vi "Write Expanded_.vi"(8 "error in (no error)":errorcluster, 10 "Expanded?":bool, 11 "MenuButton in":refnum<class "MenuButton.lvclass">) -> (0 "error out":errorcluster, 3 "MenuButton out":refnum<class "MenuButton.lvclass">)   [LabVIEW 2017, in "MenuButtons.lvlib" / "MenuButton.lvclass"]
uses:
  MenuButton.lvclass
  MenuButton.lvclass/MenuButton.ctl
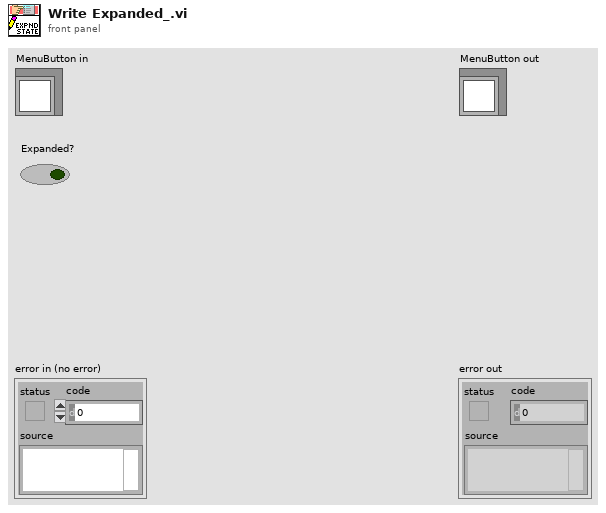
[diagram p1: front panel]
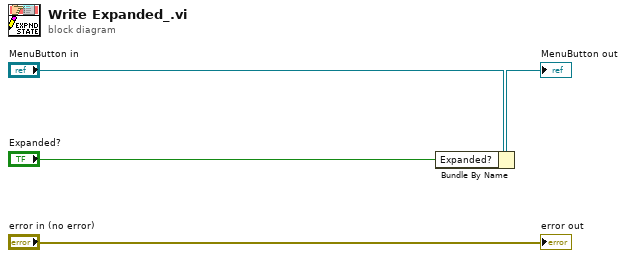
[diagram p0: block diagram]
diagram:
  n1 = Bundle By Name(cluster="MenuButton in", "Expanded?"="Expanded?") -> (→"MenuButton out":refnum<class "MenuButton.lvclass">)
  "error out" <- "error in (no error)"
